vi "Read Multiple - Wait On First Value.vi"(8 "error in (no error)":errorcluster, 9 "timeout in ms (60 sec)":i32=60000, 11 "Futures in":refnum<class "Future.lvclass">[](array[class])) -> (0 "error out":errorcluster, 2 "Result value":variant, 3 "Index of First Value":i32, 4 "All Timed Out or Errors":bool)   [LabVIEW 2017, in "Futures.lvlib" / "Future.lvclass"]
doc: "Read the result of the future.\n\nIf the future is resolved then the future becomes invalidated and cannot be read again.\n\nIf the future times out then you can attempt another read."
uses:
  Future.lvclass
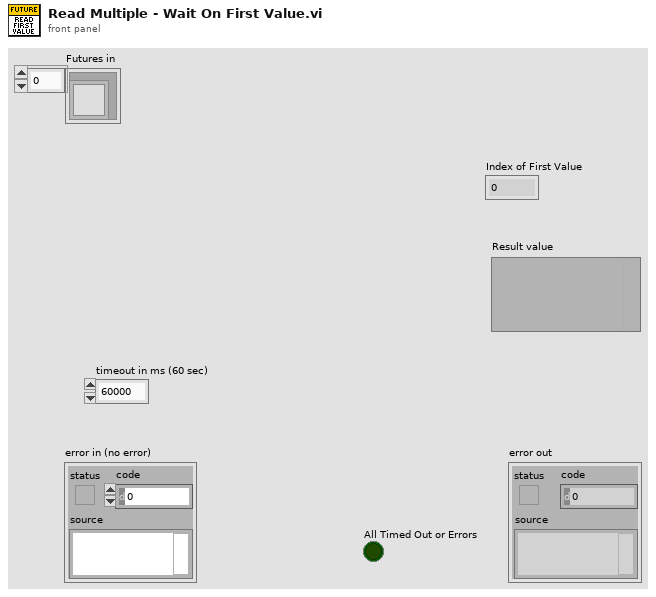
[diagram p1: front panel]
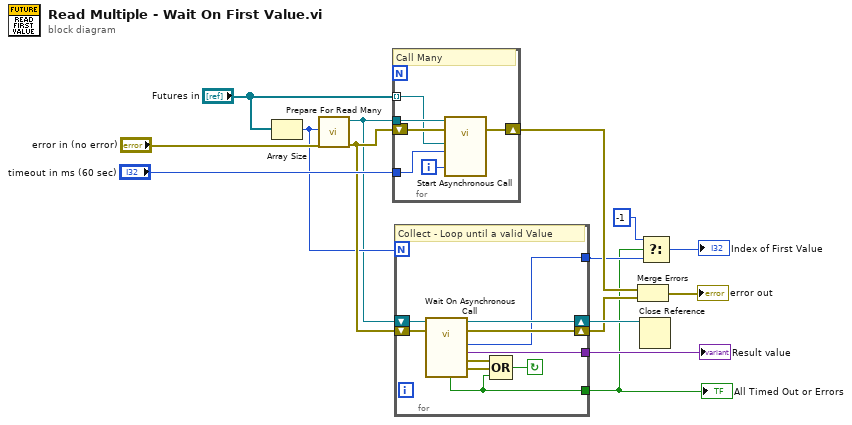
[diagram p0: block diagram]
diagram:
  n1 = Array Size(array="Futures in") -> (size(s)=w11:i32)
  n2 = call "Prepare For Read Many.vi"("error in (no error)"="error in (no error)", "Minimum Call Pool Size"=w11) -> ("error out"=w12:errorcluster, "VI out"=w10:refnum<vi>)  [unwired: 8 in]
  n3 = for {
    tunnel: w10 -> [w21]
    tunnel: "Futures in" -> [w16] mode=indexing
    shift-right: [w19] -> w7
    shift-left: w12 -> [w20]
    tunnel: "timeout in ms (60 sec)" -> [w17]
    i -> [w18]
    # "Call Many"
    n4 = call-by-ref "Start Asynchronous Call"(reference=w21, error in=w20, "Index In"=w18, "timeout in ms (60 sec)"=w17, "Future in"=w16) -> (error out=w19:errorcluster)  [unwired: 4 in, 6 out]
  }
  n5 = for {
    N: w11 -> [_]
    shift-right: [w30] -> w8
    shift-left: w12 -> [w31]
    shift-right: [w28] -> w9
    shift-left: w10 -> [w29]
    tunnel: [w25] -> w2
    tunnel: [w23] -> w5
    tunnel: [w22] -> w4
    stop <- w24 continue-if-true
    # "Collect - Loop until a valid Value"
    n6 = call-by-ref "Wait On Asynchronous Call"(reference=w29, error in=w31) -> (reference out=w28:refnum<vi>, error out=w30:errorcluster, 0:"error out"=w26:errorcluster, "Result Error"=w27:errorcluster, "Result Value"=w23:variant, "Index Out"=w22:i32, "Timed Out"=w25:bool)  [unwired: 7 in]
    n7 = Compound Arithmetic op=OR(w27, w26, w25) -> (w24:bool)
  }
  "Result value" <- w5
  "All Timed Out or Errors" <- w2
  n8 = Merge Errors(w7, w8) -> (→"error out":errorcluster)
  n9 = Close Reference(reference=w9) -> ()  [unwired: 1 in, 1 out]
  n10 = Select(t=-1, s=w2, f=w4) -> (s? t:f=→"Index of First Value":i32)
